vi "WaitListener.vi"(8 "error in (no error)":errorcluster, 11 "WebSocket in":refnum<class "WebSocket.lvclass">) -> (0 "error out":errorcluster, 3 "WebSocket out":refnum<class "WebSocket.lvclass">)   [LabVIEW 2021, in "WebSocket.lvlib" / "WebSocket.lvclass"]
uses:
  WebSocket.lvclass
  C:/Program Files (x86)/National Instruments/LabVIEW 2021/vi.lib/ActorFramework/Actor/Actor.lvclass
  WebSocket.lvclass/WebSocket.ctl
  <vilib>/MediaMongrels Ltd/WebSockets/WebSockets/WebSocket Server/WebSocket Server.lvclass
  <vilib>/ActorFramework/Actor/Actor.lvclass/Actor.ctl
  <vilib>/ActorFramework/Message Enqueuer/Message Enqueuer.lvclass/Message Enqueuer.ctl
  <vilib>/ActorFramework/Message Enqueuer/Init from Existing Queue.vi
  <vilib>/ActorFramework/Message Enqueuer/Enqueue.vi
  WebSocket Messages/Read Msg/Read Msg.lvclass
  C:/Program Files (x86)/National Instruments/LabVIEW 2021/vi.lib/ActorFramework/Message/Message.lvclass
  WebSocket Messages/WaitListener Msg/WaitListener Msg.lvclass
  <vilib>/ActorFramework/Message Priority Queue/Priority Enqueue.vi
  <vilib>/ActorFramework/Message Enqueuer/Message Enqueuer.lvclass
  <vilib>/MediaMongrels Ltd/WebSockets/Sockets/VISA TCP Listener/VISA TCP Listener.lvclass
  <vilib>/ActorFramework/Actor/Actor.lvclass
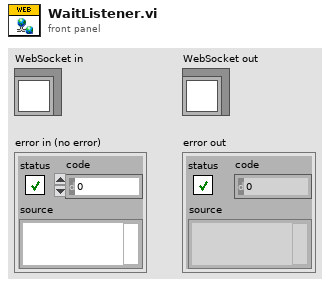
[diagram p1: front panel]
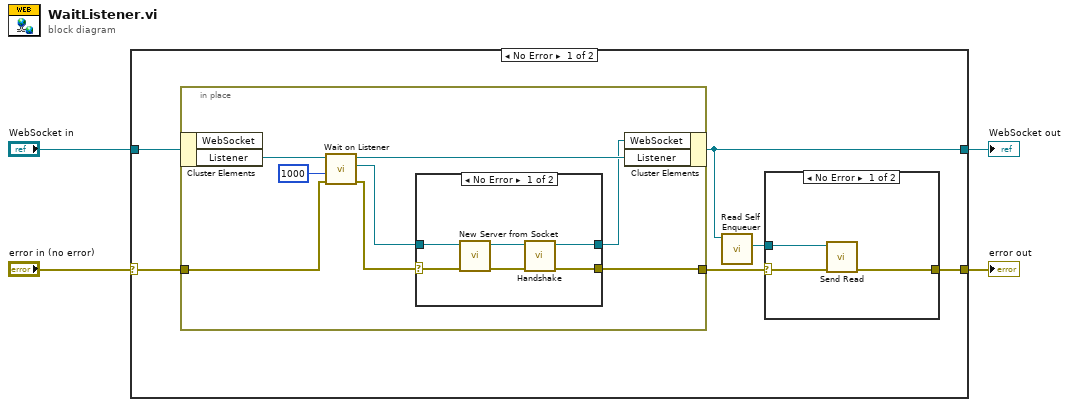
[diagram p0: block diagram]
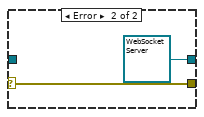
[diagram p2: hidden frame]
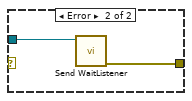
[diagram p3: hidden frame]
diagram:
  n1 = case shown="No Error" "error in (no error)" {
    selector: "error in (no error)" -> [w9 w33]
    tunnel: [w7 w33] -> w3
    tunnel: [w6 w32] -> w1
    tunnel: "WebSocket in" -> [w10 w32]
    frame No Error {
      n2 = in-place {
        in-place-border: w9 -> [w15]
        in-place-border: [w12] -> w8
        n3 = in-place-cluster #1(w10) -> ("Listener"=w18:refnum<class "VISA TCP Listener.lvclass">)  [unwired: 1 out]
        n4 = call-dynamic "Wait on Listener.vi"("error in (no error)"=w15, "timeout ms (5000)"=1000, "VISA TCP Listener in"=w18) -> ("error out"=w14:errorcluster, "Socket out"=w13:refnum<class "Socket.lvclass">, "VISA TCP Listener out"=w17:refnum<class "VISA TCP Listener.lvclass">)  [unwired: 6 in]
        n5 = case shown="No Error" w14 {
          selector: w14 -> [w21 w26]
          tunnel: w13 -> [w22 _]
          tunnel: [w20 w26] -> w12
          tunnel: [w19 refnum<class "WebSocket Server.lvclass"> refnum ("WebSocket Connection out")] -> w11
          frame No Error {
            n6 = call <vilib>:"New Server from Socket.vi"("error in (no error)"=w21, "Socket"=w22) -> ("error out"=w23:errorcluster, "WebSocket Server out"=w24:refnum<class "WebSocket Server.lvclass">)  [unwired: 8 in]
            n7 = call-dynamic "Handshake.vi"("error in (no error)"=w23, "WebSocket Connection in"=w24) -> ("error out"=w20:errorcluster, "WebSocket Connection out"=w19:refnum<class "WebSocket Server.lvclass">)  [unwired: 8 in]
          }
          frame Error {
          }
        }
        n8 = in-place-cluster #1("WebSocket"=w11, "Listener"=w17) -> (w6:refnum<class "WebSocket.lvclass">)
      }
      n9 = call <vilib>:"Read Self Enqueuer.vi"("Actor"=w6) -> ("Self Enqueuer"=w5:refnum<class "Message Enqueuer.lvclass">)  [unwired: 10 in]
      n10 = case shown="No Error" w8 {
        selector: w8 -> [w28 _]
        tunnel: [w27 w30] -> w7
        tunnel: w5 -> [w29 w31]
        frame No Error {
          n11 = call "Send Read.vi"("error in (no error)"=w28, "Message Enqueuer"=w29) -> ("error out"=w27:errorcluster)  [unwired: 8 in, 1 out]
        }
        frame Error {
          n12 = call "Send WaitListener.vi"("Message Enqueuer"=w31) -> ("error out"=w30:errorcluster)  [unwired: 9 in, 1 out]
        }
      }
    }
    frame Error {
    }
  }
  "error out" <- w3
  "WebSocket out" <- w1
